vi "WriteLogFile.vi"(6 "Automatic warning":string caption="Automatic warning (e.g. large Temperature/RH fluctuations)", 7 "Data File":string, 8 "Error In":errorcluster, 9 "DUT passed?":bool, 10 "Value TechSpec criteria":dbl, 11 "Files saved?":bool) -> (0 "Error Out":errorcluster)   [LabVIEW 2018]
uses:
  globals/QC_RunInformation.vi
panel:
  out "Cause for quitting measurement":string
  in  "OK Button":bool
  in  "Add comment":bool
  out "Type of measurement":string
  out "Logfile entry":string
  # "Write Logfile"
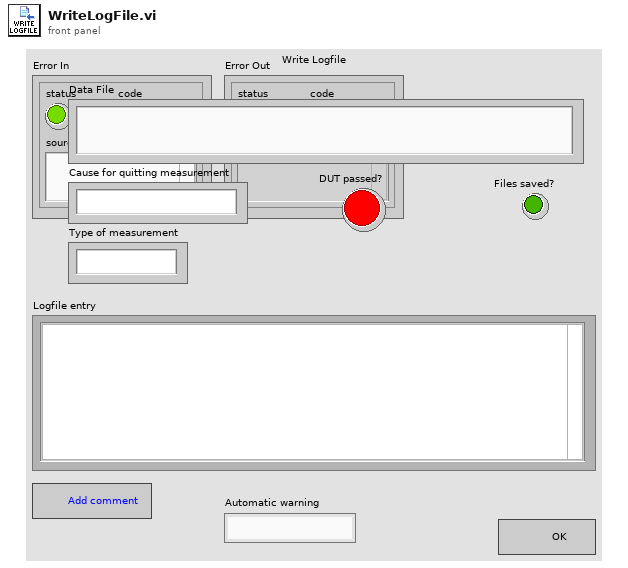
[diagram p1: front panel]
types:
  T1 = enum16{"open", "replace", "create", "open or create", "replace or create", "replace or create with confirmation"}
  T2 = cluster{"Sensor Serial No.:":string, "Wafer Serial No.:":string, "Batch:":string, "Manufacturer:":string, "Device Category:":string, "Database Serial No.:":string, "Initiated:":string, "Test":string, "Instruments used:":string, "Probeplan used:":string, "End of Run comment:":string, "User:":string}
  T3 = cluster{"Institute":string, "Manufacturers":string[], "Devices":string[], "Serialnumbers Lookup DB":string, "Data directory":string, "Backup & screenshot directory":string, "List of known users":string[]}
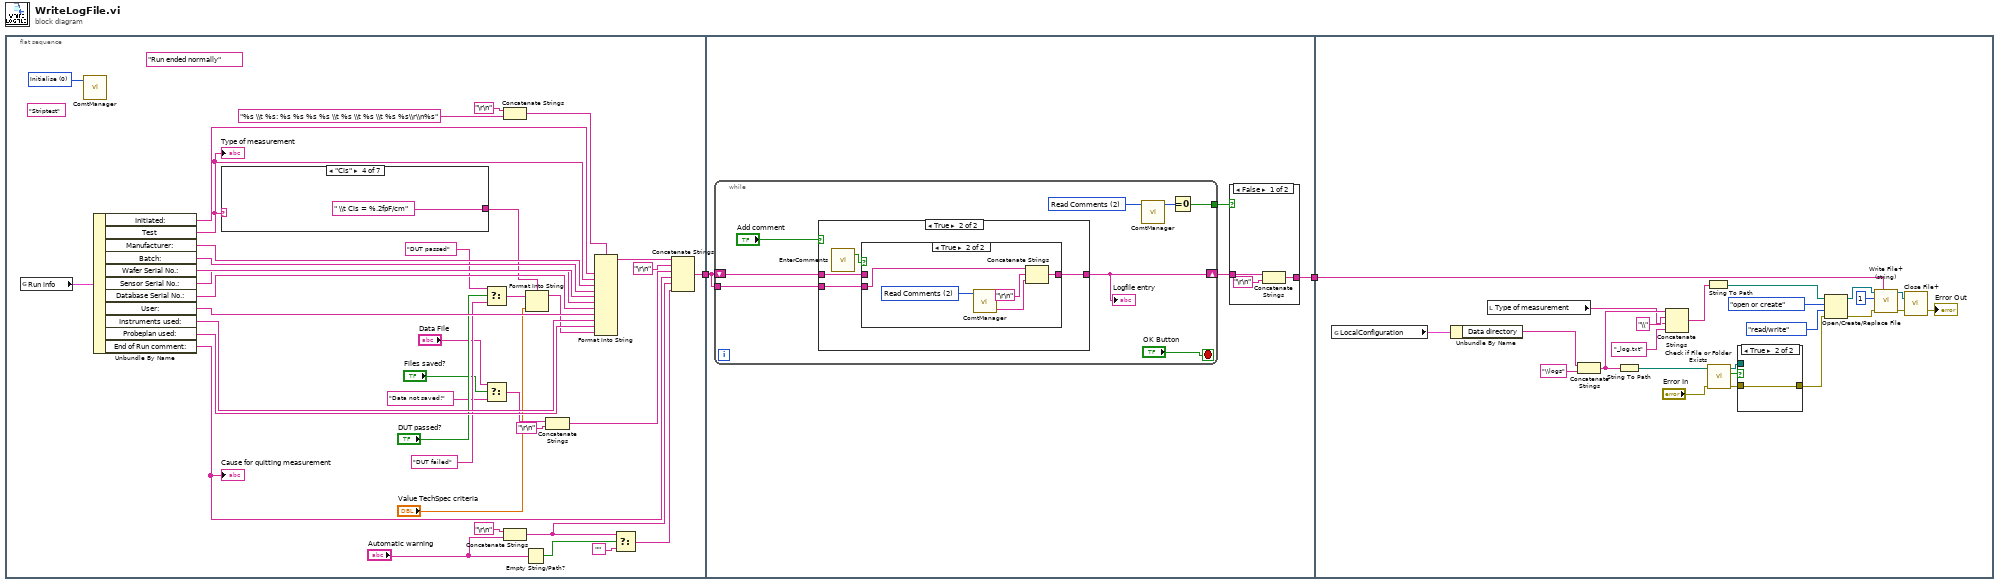
[diagram p0: block diagram]
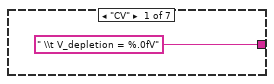
[diagram p2: hidden frame]
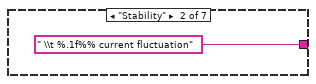
[diagram p3: hidden frame]
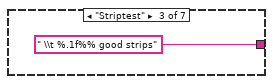
[diagram p4: hidden frame]
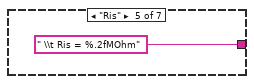
[diagram p5: hidden frame]
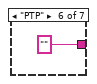
[diagram p6: hidden frame]
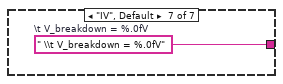
[diagram p7: hidden frame]
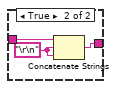
[diagram p8: hidden frame]
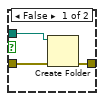
[diagram p11: hidden frame]
diagram:
  n1 = flat-sequence {
    tunnel: [w34] -> w2
    tunnel: w2 -> [w51]
    tunnel: [w49] -> w1
    tunnel: w1 -> [w92]
    frame #0 {
      (unwired) "Run ended normally" ("Cause for quitting measurement")
      (unwired) "Striptest"
      w33 = u16 0 items=["Initialise", "Add comment", "Read Comments"] ("Action")
      n2 = global read "QC_RunInformation.vi" "Run info"() -> (w32:T2)
      n3 = call "ComtManager.vi"("Action"=w33) -> ()  [unwired: 2 in, 3 out]
      n4 = Unbundle By Name(w32) -> ("Initiated:"=w40:string, "Test"=w12:string, "Manufacturer:"=w30:string, "Batch:"=w29:string, "Wafer Serial No.:"=w28:string, "Sensor Serial No.:"=w27:string, "Database Serial No.:"=w26:string, "User:"=w25:string, "Instruments used:"=w24:string, "Probeplan used:"=w23:string, "End of Run comment:"=w14:string)
      "Type of measurement" <- w12
      "Cause for quitting measurement" <- w14
      n5 = case shown="\"Cis\"" w12 {
        tunnel: [" \\t V_depletion = %.0fV" " \\t %.1f%% current fluctuation" " \\t %.1f%% good strips" " \\t Cis = %.2fpF/cm" " \\t Ris = %.2fMOhm" "" w47] -> w11
        frame "CV" {
        }
        frame "Stability" {
        }
        frame "Striptest" {
        }
        frame "Cis" {
        }
        frame "Ris" {
        }
        frame "PTP" {
        }
        frame "IV", Default {
          w47 = " \\t V_breakdown = %.0fV"  # \t V_breakdown = %.0fV
        }
      }
      n6 = Select(t="DUT passed", s="DUT passed?", f="DUT failed") -> (s? t:f=w10:string)
      n7 = Select(t="Data File", s="Files saved?", f="Data not saved!") -> (s? t:f=w16:string)
      n8 = Concatenate Strings("\r\n", "%s \\t %s: %s %s %s %s \\t %s \\t %s \\t %s %s\\r\\n%s") -> (w38:string)
      n9 = Concatenate Strings("\r\n", "Automatic warning") -> (w5:string)
      n10 = Empty String/Path?(string/path="Automatic warning") -> (empty?=w7:bool)
      n11 = Format Into String(format string=w11, initial string=w10, "Value TechSpec criteria") -> (resulting string=w9:string)  [unwired: 1 in, 1 out]
      n12 = Concatenate Strings(w16, "\r\n") -> (w35:string)
      n13 = Format Into String(format string=w38, w40, w12, w30, w29, w28, w27, w26, w25, w24, w23, w9) -> (resulting string=w36:string)  [unwired: 2 in, 1 out]
      n14 = Select(t=w5, s=w7, f="") -> (s? t:f=w3:string)
      n15 = Concatenate Strings(w36, "\r\n", w35, w14, w5, w3) -> (w34:string)
    }
    frame #1 {
      n16 = while {
        shift-right: [w61] -> w50
        shift-left: w51 -> [w63]
        tunnel: w51 -> [w62]
        tunnel: [w58] -> w48
        stop <- "OK Button" stop-if-true
        w60 = u16 2 items=["Initialise", "Add comment", "Read Comments"] ("Action")
        n17 = case shown="True" "Add comment" {
          tunnel: [w66 w69] -> w61
          tunnel: w63 -> [w66 w68]
          tunnel: w62 -> [_ w67]
          frame False {
          }
          frame True {
            n18 = call "EnterComments.vi"() -> ("update?"=w70:bool)  [unwired: 4 in]
            n19 = case shown="True" w70 {
              tunnel: [w71 w75] -> w69
              tunnel: w68 -> [w71 _]
              tunnel: w67 -> [_ w74]
              frame False {
              }
              frame True {
                w76 = u16 2 items=["Initialise", "Add comment", "Read Comments"] ("Action")
                n20 = call "ComtManager.vi"("Action"=w76) -> ("Comment out"=w73:string)  [unwired: 2 in, 2 out]
                n21 = Concatenate Strings(w74, "\r\n", w73) -> (w75:string)
              }
            }
          }
        }
        "Logfile entry" <- w61
        n22 = call "ComtManager.vi"("Action"=w60) -> ("No of comments"=w59:i32)  [unwired: 2 in, 2 out]
        n23 = Equal To 0?(x=w59) -> (x = 0?=w58:bool)
      }
      n24 = case shown="False" w48 {
        tunnel: w50 -> [w53 w55]
        tunnel: [w52 w56] -> w49
        frame False {
          n25 = Concatenate Strings(w53, "\r\n") -> (w52:string)
        }
        frame True {
          w57 = "\r\n"
          n26 = Concatenate Strings(w55, w57, w57) -> (w56:string)
        }
      }
    }
    frame #2 {
      n27 = global read "QC_RunInformation.vi" "LocalConfiguration"() -> (w91:T3)
      n28 = Unbundle By Name(w91) -> ("Data directory"=w89:string)
      n29 = local read "Type of measurement"() -> (w77:string)
      n30 = Concatenate Strings(w89, "\\logs") -> (w86:string)
      n31 = String To Path(string=w86) -> (path=w83:path)
      n32 = Concatenate Strings(w86, "\\", w77, "_log.txt") -> (w85:string)
      n33 = String To Path(string=w85) -> (path=w84:path)
      n34 = call <vilib>:"Check if File or Folder Exists.vi"("error in (no error)"="Error In", "path"=w83) -> ("error out"=w79:errorcluster, "file or folder exists?"=w82:bool, "dup path"=w81:path)  [unwired: 7 in]
      n35 = case shown="True" w82 {
        tunnel: w81 -> [w103 _]
        tunnel: w79 -> [w102 w104]
        tunnel: [w101 w104] -> w78
        frame False {
          n36 = Create Folder(path (use dialog)=w103, error in=w102) -> (error out=w101:errorcluster)  [unwired: 1 in, 2 out]
        }
        frame True {
        }
      }
      n37 = Open/Create/Replace File(file path (use dialog)=w84, error in=w78, operation (0:open)=T1."open or create", access (0:read/write)=enum16{"read/write", "read-only", "write-only"}."read/write") -> (refnum out=w97:refnum<file>, error out=w98:errorcluster)  [unwired: 2 in, 1 out]
      n38 = call <vilib>:"Write File+ (string).vi"("string"=w92, "error in (no error)"=w98, "pos mode (rel. to end:1)"=1, "refnum"=w97) -> ("error out"=w94:errorcluster, "dup refnum"=w93:refnum<file>)  [unwired: 3 in, 1 out]
      n39 = call <vilib>:"Close File+.vi"("error in (no error)"=w94, "refnum"=w93) -> ("error out"=→"Error Out":errorcluster)  [unwired: 3 in, 2 out]
    }
  }
